vi "Create Folders.vi"(8 "error in (no error)":errorcluster, 11 "PostBuildSupport in":refnum<class "PostBuildSupport.lvclass">) -> (0 "error out":errorcluster, 3 "PostBuildSupport out":refnum<class "PostBuildSupport.lvclass">)   [LabVIEW 2016, in "PostBuildSupport.lvclass"]
uses:
  PostBuildSupport.lvclass
  PostBuildSupport.lvclass/PostBuildSupport.ctl
  <userlib>/_MGI/File/MGI Create Directory Chain Behavior Enum.ctl
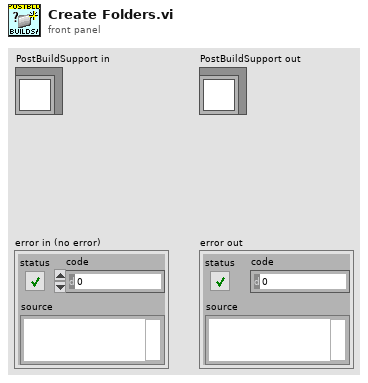
[diagram p1: front panel]
types:
  T1 = typedef "MGI Create Directory Chain Behavior Enum.ctl" = enum16{"Auto Detect", "Path Contains a File", "Path Does Not Contain a File"}
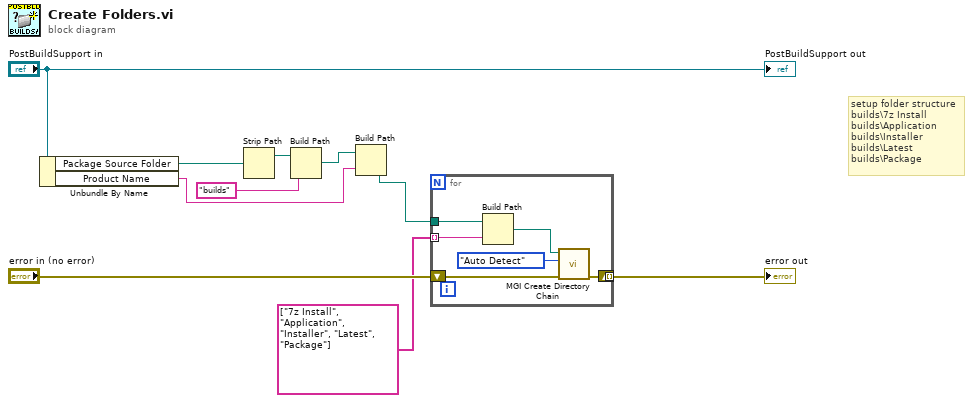
[diagram p0: block diagram]
diagram:
  # "setup folder structure\nbuilds\\7z Install\nbuilds\\Application\nbuilds\\Installer\nbuilds\\Latest\nbuilds\\Package"
  n1 = Unbundle By Name("PostBuildSupport in") -> ("Package Source Folder"=w5:path, "Product Name"=w4:string)
  n2 = Strip Path(path=w5) -> (stripped path=w3:path)  [unwired: 1 out]
  n3 = Build Path(base path=w3, name or relative path="builds") -> (appended path=w7:path)
  n4 = Build Path(base path=w7, name or relative path=w4) -> (appended path=w2:path)
  n5 = for {
    shift-right: [w11] -> w1
    shift-left: "error in (no error)" -> [w15]
    tunnel: w2 -> [w14]
    tunnel: string[] ["7z Install", "Application", "Installer", "Latest", "Package"] -> [w13] mode=indexing
    tunnel: [w11] -> _ mode=indexing
    n6 = Build Path(base path=w14, name or relative path=w13) -> (appended path=w12:path)
    n7 = call <userlib>:"MGI Create Directory Chain.vi"("Error In"=w15, "File Presence (Auto Detect)"=MGI_Create_Directory_Chain_Behavior_Enum."Auto Detect", "Path"=w12) -> ("Error Out"=w11:errorcluster)  [unwired: 7 in, 1 out]
  }
  "error out" <- w1
  "PostBuildSupport out" <- "PostBuildSupport in"
